vi "二进制文件（复杂数据读写）.vi"() -> ()   [LabVIEW 2017]
panel:
  out "波形图":dbl[](graph)
  out "大小（字节）":i64
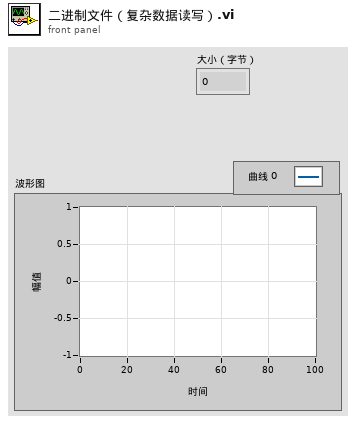
[diagram p1: front panel]
types:
  T1 = enum16{"open", "replace", "create", "open or create", "replace or create", "replace or create with confirmation"}
  T2 = cluster{"seconds since 1Jan1904":timestamp, dbl}[]
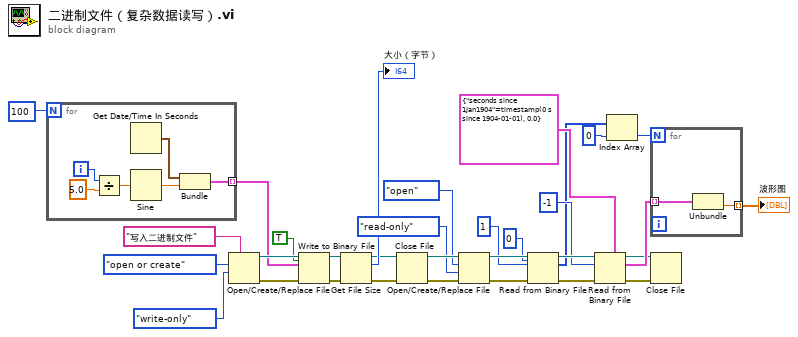
[diagram p0: block diagram]
diagram:
  n1 = for {
    N: 100 -> [_]
    tunnel: [w33] -> w25 mode=indexing
    i -> [w38]
    n2 = Divide(x=w38, y=5.0) -> (x/y=w36:dbl)
    n3 = Get Date/Time In Seconds() -> (seconds since 1Jan1904=w35:timestamp)
    n4 = Sine(x=w36) -> (sin(x)=w34:dbl)
    n5 = Bundle("seconds since 1Jan1904"=w35, w34) -> (w33:cluster{"seconds since 1Jan1904":timestamp, dbl})  [unwired: 1 in]
  }
  n6 = Open/Create/Replace File(prompt="写入二进制文件" ("提示"), operation (0:open)=T1."open or create" ("操作(0:open)"), access (0:read/write)=enum16{"read/write", "read-only", "write-only"}."write-only" ("权限(0:read/write)")) -> (refnum out=w28:refnum<file>, error out=w27:errorcluster)  [unwired: 3 in, 1 out]
  n7 = Write to Binary File(file (use dialog)=w28, data=w25, error in=w27, 5:TRUE ("预置数组或字符串大小？ (T)")) -> (refnum out=w23:refnum<file>, error out=w24:errorcluster)  [unwired: 2 in, 1 out]
  n8 = Get File Size(file=w23, error in=w24) -> (refnum out=w20:refnum<file>, size (in bytes)=→"大小（字节）":i64, 0:w21:errorcluster)
  n9 = Close File(refnum=w20, error in=w21) -> (path=w18:path, error out=w19:errorcluster)
  n10 = Open/Create/Replace File(file path (use dialog)=w18, error in=w19, operation (0:open)=T1."open" ("操作(0:open)"), access (0:read/write)=enum16{"read/write", "read-only", "write-only"}."read-only" ("权限(0:read/write)")) -> (refnum out=w14:refnum<file>, error out=w15:errorcluster)  [unwired: 2 in, 1 out]
  n11 = Read from Binary File(5:0, 8:w15, 10:1 ("总数(1)"), 11:w14) -> (0:w11:errorcluster, 2:w7:i32[], 3:w10:refnum<file>)  [unwired: 2 in, 1 out]
  n12 = Read from Binary File(5:cluster{"seconds since 1Jan1904":timestamp, dbl} {"seconds since 1Jan1904"=timestamp(0 s since 1904-01-01), 0.0} ("输出簇"), 8:w11, 10:-1 ("总数(1)"), 11:w10) -> (0:w2:errorcluster, 2:w4:T2, 3:w3:refnum<file>)  [unwired: 2 in, 1 out]
  n13 = Index Array(array=w7, index=0 ("长度")) -> (element=w5:i32)
  n14 = for {
    N: w5 -> [_]
    tunnel: w4 -> [w40] mode=indexing
    tunnel: [w39] -> w1 mode=indexing
    n15 = Unbundle(w40) -> (w39:dbl)  [unwired: 1 out]
  }
  "波形图" <- w1
  n16 = Close File(refnum=w3, error in=w2) -> ()  [unwired: 2 out]
